vi "compare two string arrays.vi"(10 "Array 2":string[](array[string]), 11 "Array 1":string[](array[string])) -> (1 "Array 2 items missing in Array 1":string[](array[string]), 3 "Boolean":bool)   [LabVIEW 2013]
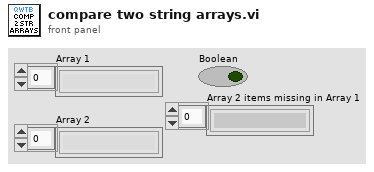
[diagram p1: front panel]
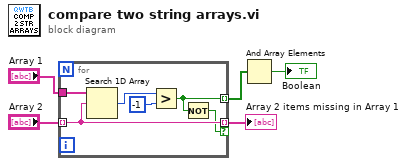
[diagram p0: block diagram]
diagram:
  n1 = for {
    tunnel: "Array 2" -> [w8] mode=indexing
    tunnel: "Array 1" -> [w11]
    tunnel: [w6] -> w2 mode=indexing
    tunnel: [w8] -> w1 mode=indexing if=w7
    n2 = Search 1D Array(1D array=w11, element=w8) -> (index of element=w10:i32)  [unwired: 1 in]
    n3 = Greater?(x=w10, y=-1) -> (0:w6:bool)
    n4 = Not(x=w6) -> (.not. x?=w7:bool)
  }
  "Array 2 items missing in Array 1" <- w1
  n5 = And Array Elements(Boolean array=w2) -> (logical AND=→"Boolean":bool)
